vi "Digital Input Convert Data to JSON string.vi"(8 "error in":errorcluster, 10 "DIO Configuration":T1[](array[typedef]), 11 "Data In":bool[](array[boolean])) -> (0 "error out":errorcluster, 3 "JSON String":string)   [LabVIEW 2024]
doc: "All Rights Reserved © 2017 SyncSols"
uses:
  Digital Output/SubVIs/Digital Dynamic Cluster.ctl
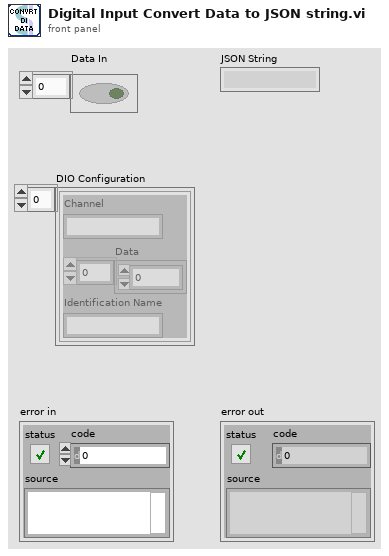
[diagram p1: front panel]
types:
  T1 = typedef "Digital Dynamic Cluster.ctl" = cluster{"Channel":string, "Data":u8[], "Identification Name":string}
  T2 = cluster{"Command":string, "SubCmd":string, "Channels":string[], "Data":i16[], "Time":string}
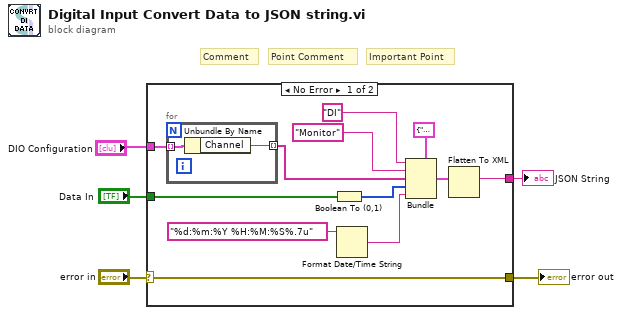
[diagram p0: block diagram]
diagram:
  # "Important Point"
  # "Point Comment"
  # "Comment"
  n1 = case shown="No Error" "error in" {
    selector: "error in" -> [w6 w20]
    tunnel: [w6 w20] -> w5
    tunnel: "Data In" -> [w17 _]
    tunnel: [w7 _] -> w2
    tunnel: "DIO Configuration" -> [w14 _]
    frame No Error {
      n2 = for {
        tunnel: w14 -> [w19] mode=indexing
        tunnel: [w18] -> w12 mode=indexing
        n3 = Unbundle By Name(w19) -> ("Channel"=w18:string)
      }
      n4 = Boolean To (0,1)(Boolean=w17) -> (0, 1=w13:i16[])
      n5 = Format Date/Time String(time format string (%c)="%d:%m:%Y %H:%M:%S%.7u") -> (date/time string=w9:string)  [unwired: 2 in]
      n6 = Bundle(cluster=T2 {"Command"="", "SubCmd"="", "Channels"=[], "Data"=[], "Time"=""}, "Command"="DI", "SubCmd"="Monitor" ("Sub Cmd"), "Channels"=w12, "Data"=w13, "Time"=w9) -> (w8:T2)
      n7 = Flatten To XML(anything=w8) -> (xml string=w7:string)
    }
    frame Error {
    }
  }
  "error out" <- w5
  "JSON String" <- w2
